vi "Close.vi"(8 "error in (no error)":errorcluster, 11 "ChromaAcLoad in":refnum<class "ChromaAcLoad.lvclass">) -> (0 "error out":errorcluster, 3 "ChromaAcLoad out":refnum<class "ChromaAcLoad.lvclass">)   [LabVIEW 2018, in "AcPwrPlugins.lvlib" / "ChromaAcLoad.lvclass"]
doc: "This VI closes the reference to the instrument(s)."
uses:
  ChromaAcLoad.lvclass
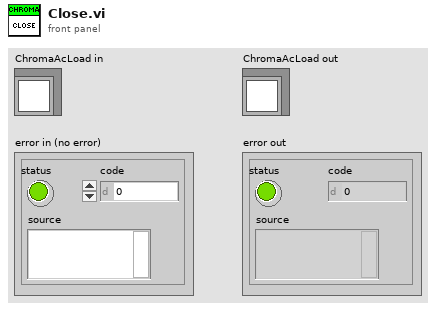
[diagram p1: front panel]
types:
  T1 = typedef "AcPwrPlugins.lvlib/ChromaAcLoad.lvclass/DeviceProperties.ctl" = cluster{"Configuration Mode":enum16{"Constant Voltage (DC)", "Constant Power (DC)", "Constant Power (AC)", "Constant Current (DC)", "Constant Current (AC)", "Constant Resistance (DC)", "Constant Resistance (AC)", "Rectified Mode (DC)", "Inrush (AC)", "RLC CP (AC)", "RLC (AC)"}, "Phases":cluster{"Handle":string, "Name":string, "Phase Select":i32, "Instrument Options":string, "id query (T)":bool, "reset device (T)":bool, "Load Short Circuited":bool, "Line Synchronization":bool, "Load Current (A/Arms)":dbl, "Load Voltage (V/Vrms)":dbl, "Load Power (W)":dbl, "Load Resistance (Ohms)":dbl, "Load Current Peak Limit (A)":dbl, "Load Current Limit (A/Arms)":dbl, "Load Power Limit (W)":dbl, "Synch Frequency (Hz)":dbl, "Priority":enum16{"CF Only", "PF Only", "Both (CF)", "Both (PF)"}, "Crest Factor":dbl, "Power Factor":dbl, "Slew Rate":cluster{"Rise Slew Rate (A/ms)":i32, "Fall Slew Rate (A/ms)":i32}, "LC/RLC Mode":cluster{"Capacitance (uF)":i32, "Inductance (uH)":i32, "Series Resistance (Ohm)":dbl, "Parallel Resistance (Ohm)":dbl}, "Timing":cluster{"TimingOn":enum16{""}, "Hours":u32, "Minutes":u32, "Seconds":dbl, "CutoffVoltage":dbl}, "Connected":bool}[]}
  T2 = cluster{"Handle":string, "Name":string, "Phase Select":i32, "Instrument Options":string, "id query (T)":bool, "reset device (T)":bool, "Load Short Circuited":bool, "Line Synchronization":bool, "Load Current (A/Arms)":dbl, "Load Voltage (V/Vrms)":dbl, "Load Power (W)":dbl, "Load Resistance (Ohms)":dbl, "Load Current Peak Limit (A)":dbl, "Load Current Limit (A/Arms)":dbl, "Load Power Limit (W)":dbl, "Synch Frequency (Hz)":dbl, "Priority":enum16{"CF Only", "PF Only", "Both (CF)", "Both (PF)"}, "Crest Factor":dbl, "Power Factor":dbl, "Slew Rate":cluster{"Rise Slew Rate (A/ms)":i32, "Fall Slew Rate (A/ms)":i32}, "LC/RLC Mode":cluster{"Capacitance (uF)":i32, "Inductance (uH)":i32, "Series Resistance (Ohm)":dbl, "Parallel Resistance (Ohm)":dbl}, "Timing":cluster{"TimingOn":enum16{""}, "Hours":u32, "Minutes":u32, "Seconds":dbl, "CutoffVoltage":dbl}, "Connected":bool}[]
  T3 = cluster{"Handle":string, "Name":string, "Phase Select":i32, "Instrument Options":string, "id query (T)":bool, "reset device (T)":bool, "Load Short Circuited":bool, "Line Synchronization":bool, "Load Current (A/Arms)":dbl, "Load Voltage (V/Vrms)":dbl, "Load Power (W)":dbl, "Load Resistance (Ohms)":dbl, "Load Current Peak Limit (A)":dbl, "Load Current Limit (A/Arms)":dbl, "Load Power Limit (W)":dbl, "Synch Frequency (Hz)":dbl, "Priority":enum16{"CF Only", "PF Only", "Both (CF)", "Both (PF)"}, "Crest Factor":dbl, "Power Factor":dbl, "Slew Rate":cluster{"Rise Slew Rate (A/ms)":i32, "Fall Slew Rate (A/ms)":i32}, "LC/RLC Mode":cluster{"Capacitance (uF)":i32, "Inductance (uH)":i32, "Series Resistance (Ohm)":dbl, "Parallel Resistance (Ohm)":dbl}, "Timing":cluster{"TimingOn":enum16{""}, "Hours":u32, "Minutes":u32, "Seconds":dbl, "CutoffVoltage":dbl}, "Connected":bool}
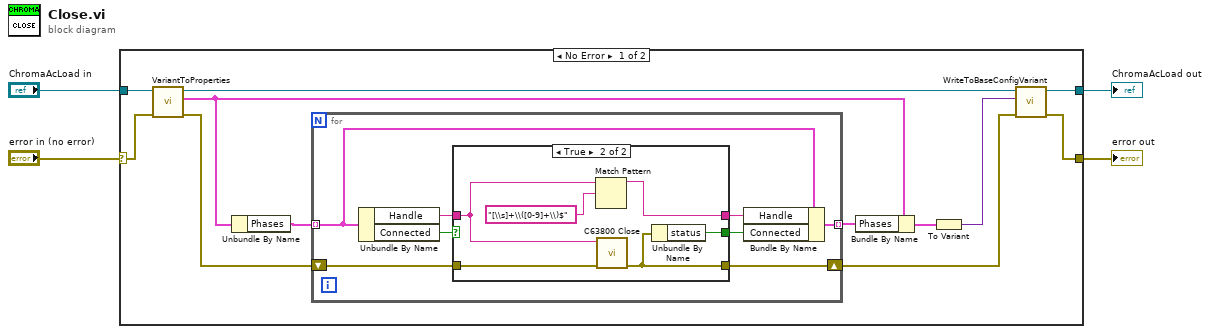
[diagram p0: block diagram]
diagram:
  n1 = case shown="No Error" "error in (no error)" {
    selector: "error in (no error)" -> [w15 w34]
    tunnel: [w5 w35] -> w4
    tunnel: "ChromaAcLoad in" -> [w16 w35]
    tunnel: [w8 w34] -> w1
    frame No Error {
      n2 = call "VariantToProperties.vi"("error in (no error)"=w15, "ChromaAcLoad"=w16) -> ("error out"=w12:errorcluster, "Device Properties"=w10:T1, "ChromaAcLoad"=w6:refnum<class "ChromaAcLoad.lvclass">)  [unwired: 7 in]
      n3 = Unbundle By Name(w10) -> ("Phases"=w14:T2)
      n4 = for {
        tunnel: w14 -> [w24] mode=indexing
        shift-right: [w22] -> w9
        shift-left: w12 -> [w23]
        tunnel: [w21] -> w13 mode=indexing
        n5 = Unbundle By Name(w24) -> ("Handle"=w20:string, "Connected"=w17:bool)
        n6 = case shown="True" w17 {
          selector: w17 -> [w25 _]
          tunnel: w20 -> [w26 w30]
          tunnel: w23 -> [w27 w31]
          tunnel: [w27 w29] -> w22
          tunnel: [w26 w32] -> w19
          tunnel: [w25 w28] -> w18
          frame False {
          }
          frame True {
            n7 = Match Pattern(string=w30, regular expression="[\\s]+\\([0-9]+\\)$") -> (before substring=w32:string)  [unwired: 1 in, 3 out]
            n8 = call <instrlib>:"C63800 Close.vi"("error in (no error)"=w31, "Instrument Handle"=w30) -> ("error out"=w29:errorcluster)  [unwired: 9 in]
            n9 = Unbundle By Name(w29) -> ("status"=w28:bool)
          }
        }
        n10 = Bundle By Name(cluster=w24, "Handle"=w19, "Connected"=w18) -> (w21:T3)
      }
      n11 = Bundle By Name(cluster=w10, "Phases"=w13) -> (w11:T1)
      n12 = To Variant(anything=w11) -> (Variant=w7:variant)
      n13 = call "WriteToBaseConfigVariant.vi"("error in (no error)"=w9, "Variant"=w7, "ChromaAcLoad in"=w6) -> ("error out"=w8:errorcluster, "ChromaAcLoad out"=w5:refnum<class "ChromaAcLoad.lvclass">)  [unwired: 7 in]
    }
    frame Error {
    }
  }
  "error out" <- w1
  "ChromaAcLoad out" <- w4
